vi "read_weather_station.vi"() -> ()   [LabVIEW 2011]
panel:
  out "Deque error":errorcluster
  out "DataSocket error":errorcluster
  out "# Sent Data":u64
  out "Solar position (elevation)":string
  out "Solar position (azimuth)":string
  out "Dew point temperature":string
  out "Absolute air humidity":string
  out "Relative air humidity":string
  out "Relative air pressure":string
  out "Absolute air pressure":string
  out "Wind direction":string
  out "Wind velocity":string
  out "Precipiation":string
  out "Outside temperature":string
  out "Global radiation":string
  out "Twilight":string
  out "Brigthness, western direction":string
  out "Brigthness, southern direction":string
  out "Brigthness, eastern direction":string
  out "Brigthness, northen direction":string
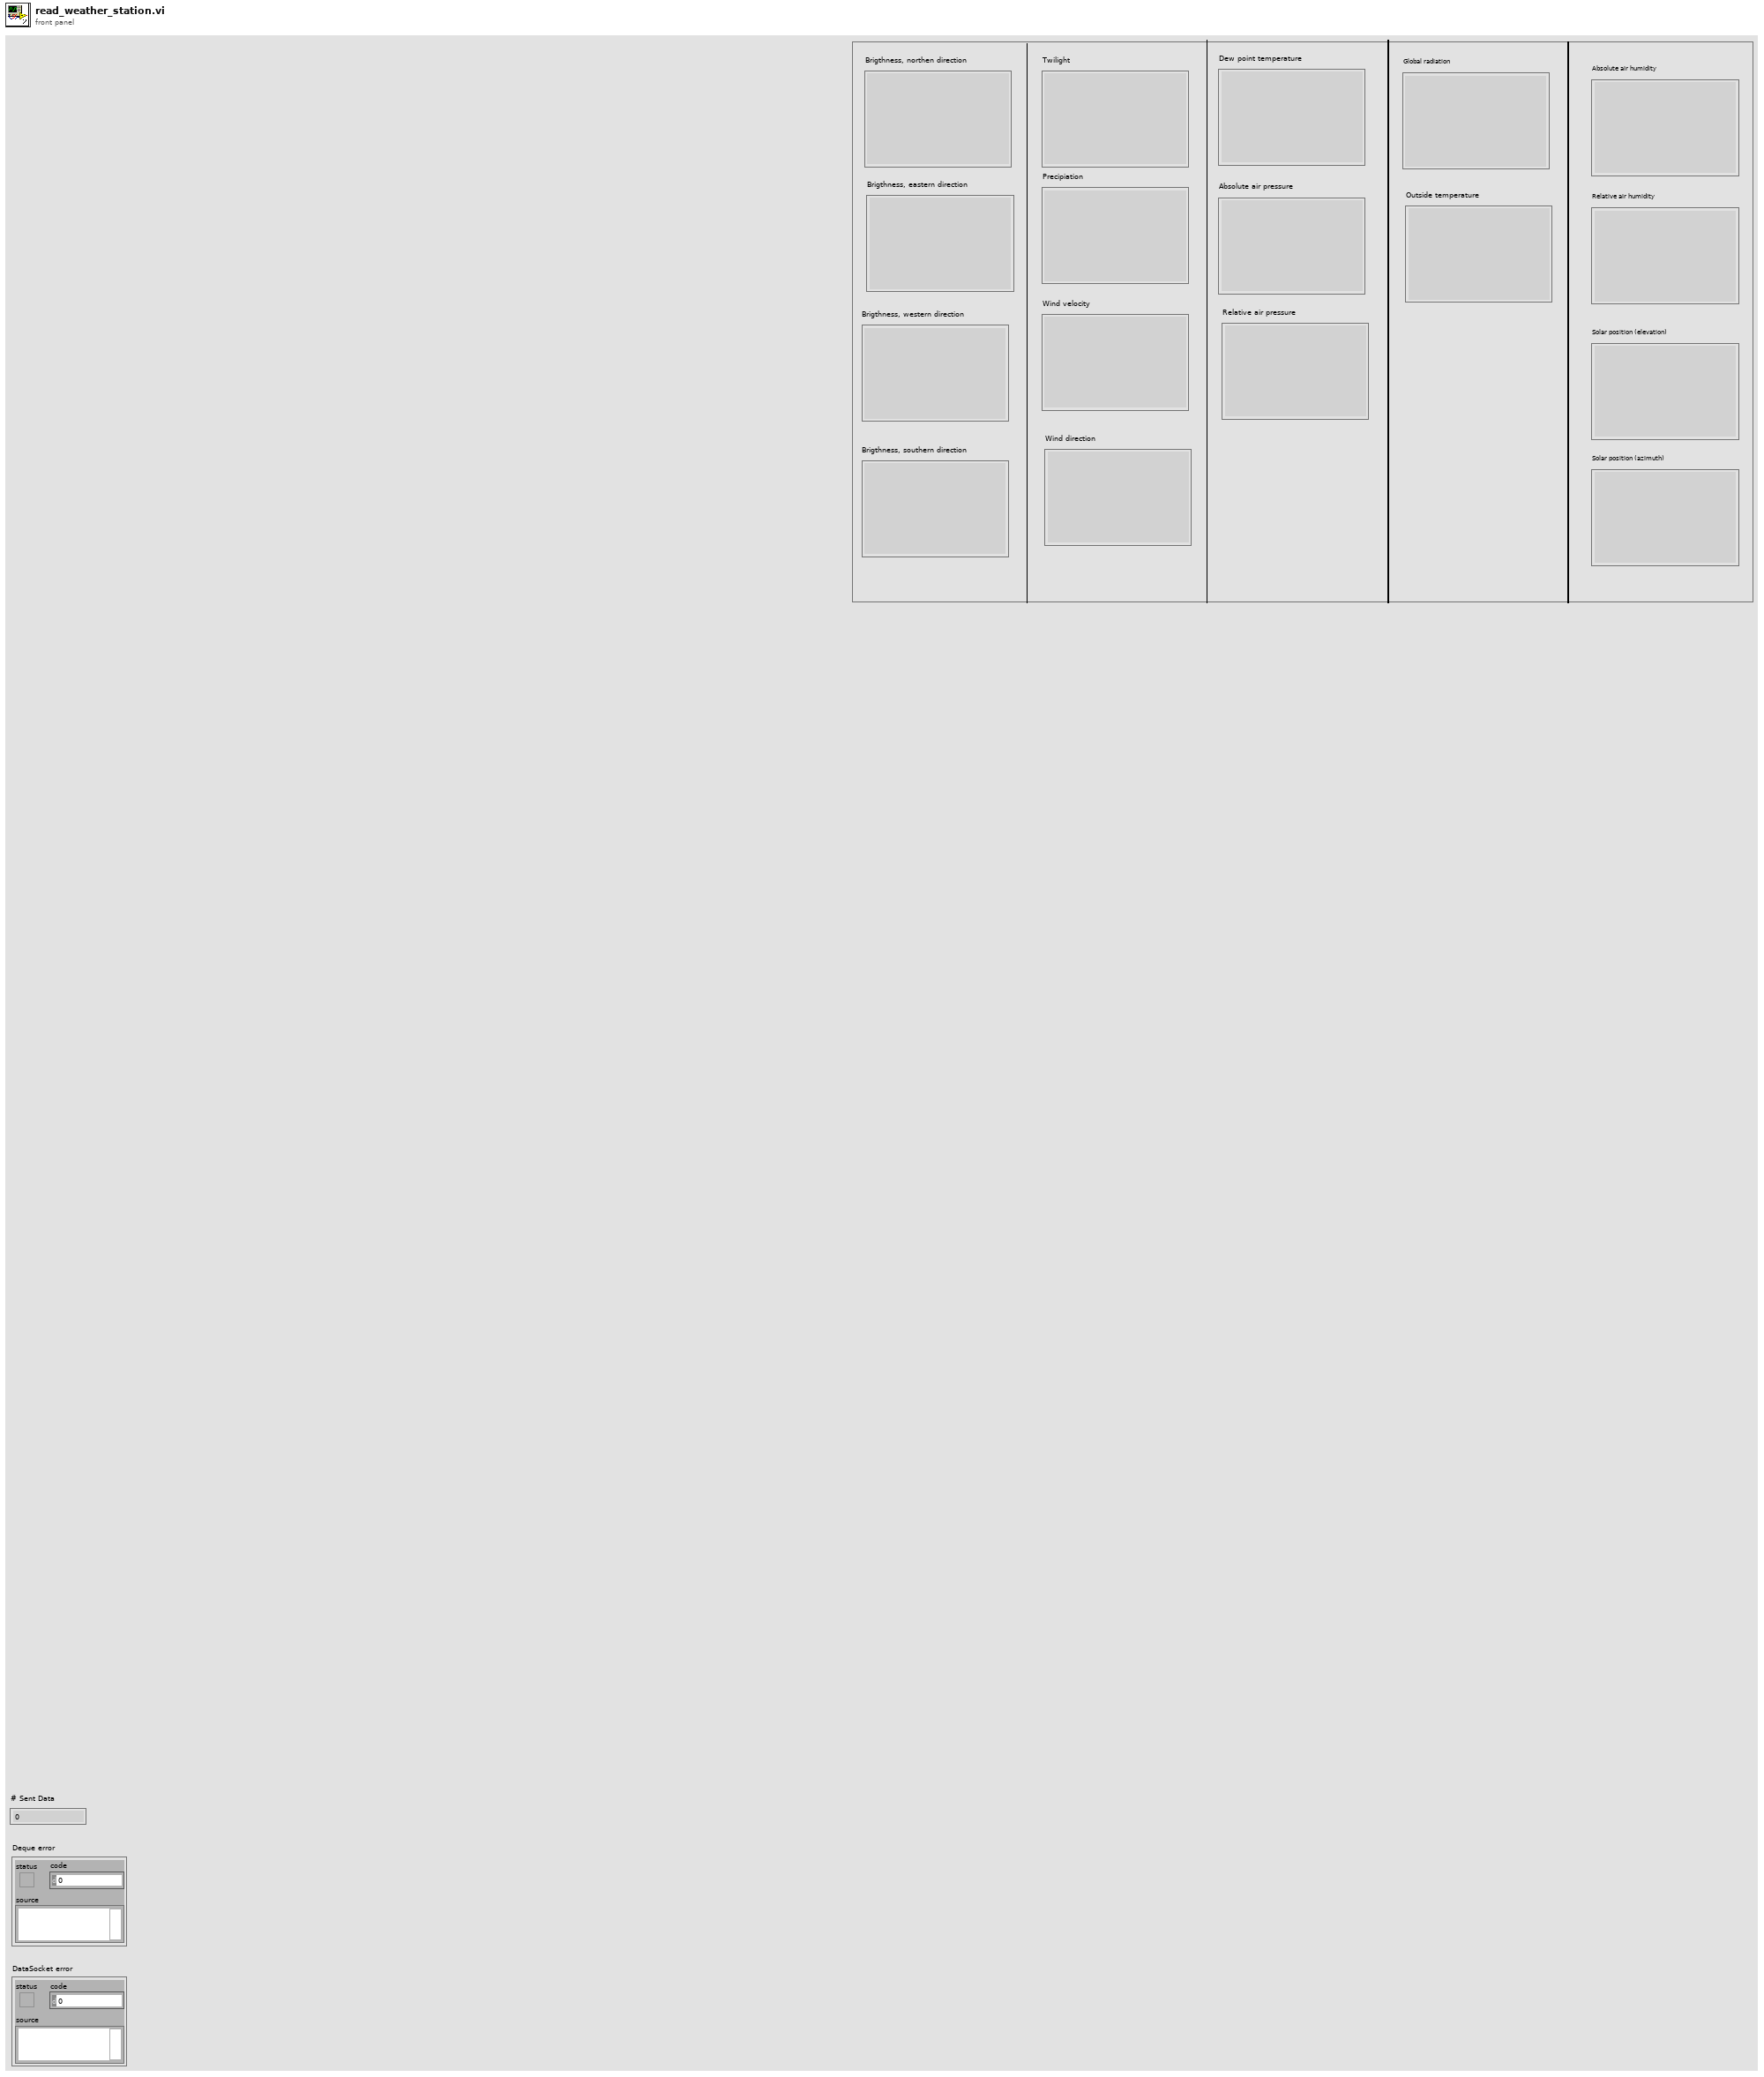
[diagram p1: front panel]
types:
  T1 = enum16{"Read", "Write", "ReadWrite", "BufferedRead", "BufferedReadWrite"}
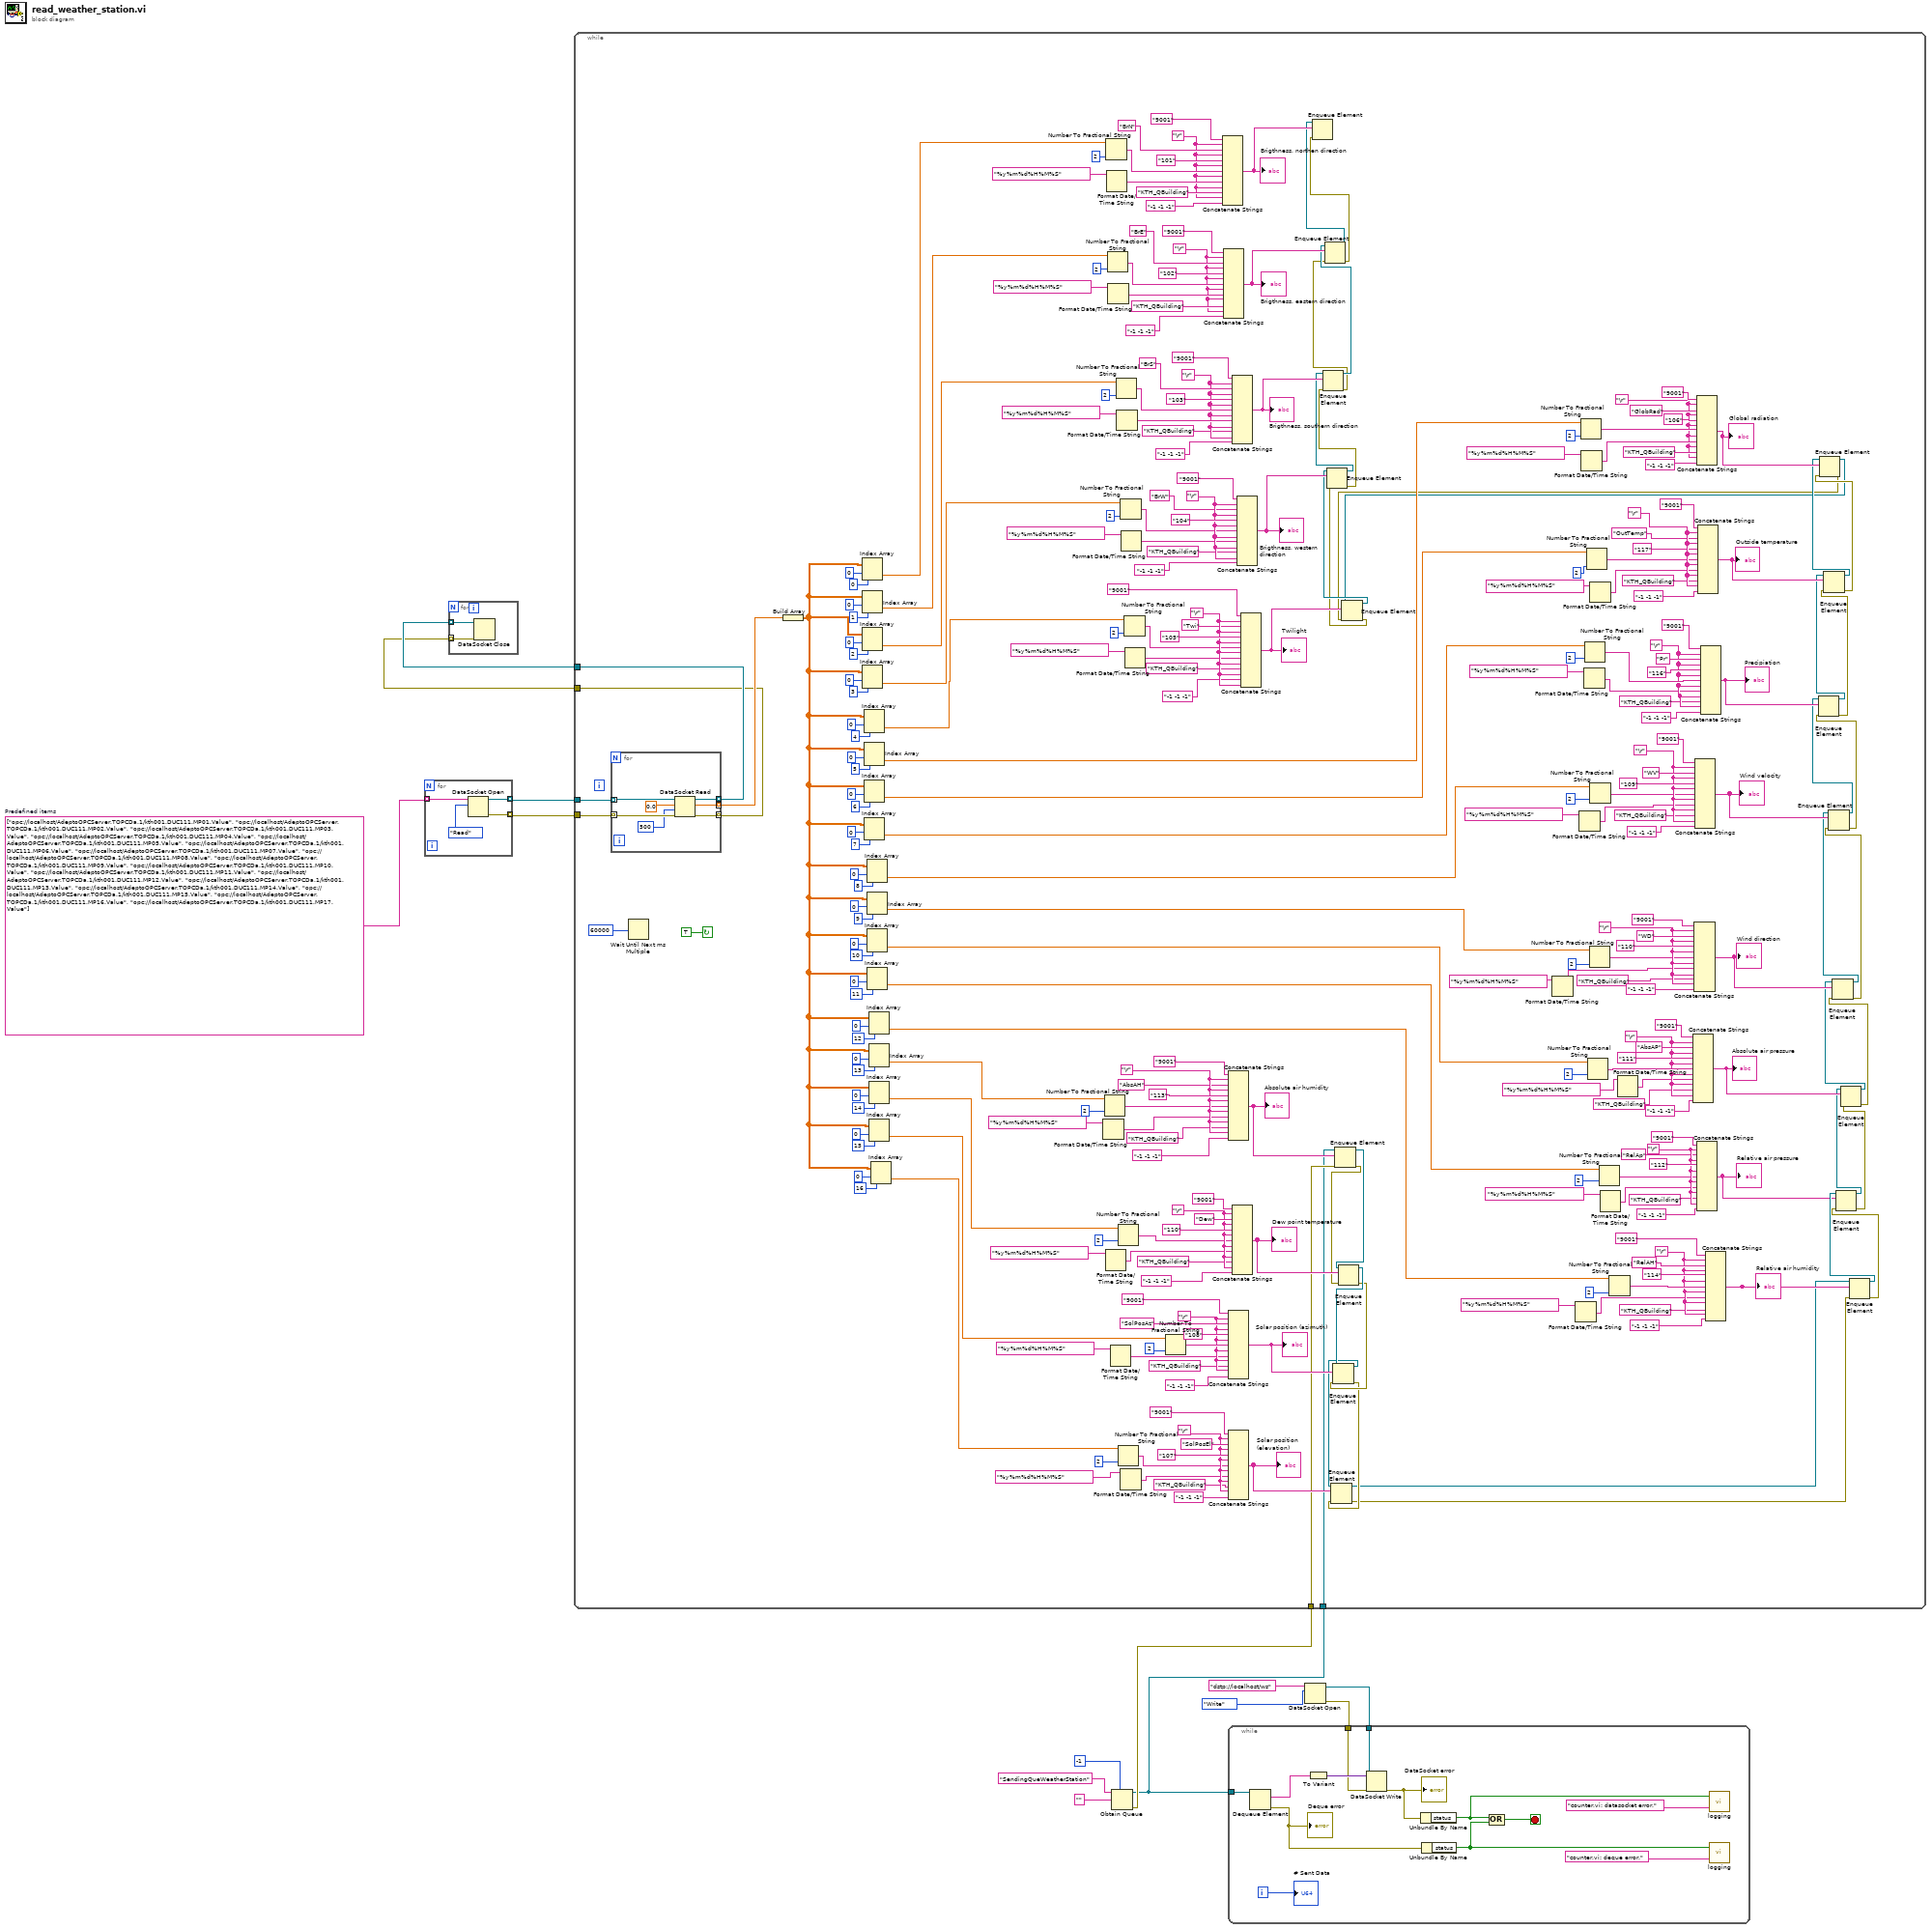
[diagram p0: block diagram]
diagram:
  w14 = string[] ["opc://localhost/AdeptoOPCServer.TOPCDa.1/kth001.DUC111.MP01.Value", "opc://localhost/AdeptoOPCServer.TOPCDa.1/kth001.DUC111.MP02.Value", "opc://localhost/AdeptoOPCServer.TOPCDa.1/kth001.DUC111.MP03.Value", "opc://localhost/AdeptoOPCServer.TOPCDa.1/kth001.DUC111.MP04.Value", "opc://localhost/AdeptoOPCServer.TOPCDa.1/kth001.DUC111.MP05.Value", "opc://localhost/AdeptoOPCServer.TOPCDa.1/kth001.DUC111.MP06.Value", "opc://localhost/AdeptoOPCServer.TOPCDa.1/kth001.DUC111.MP07.Value", "opc://localhost/AdeptoOPCServer.TOPCDa.1/kth001.DUC111.MP08.Value", "opc://localhost/AdeptoOPCServer.TOPCDa.1/kth001.DUC111.MP09.Value", "opc://localhost/AdeptoOPCServer.TOPCDa.1/kth001.DUC111.MP10.Value", "opc://localhost/AdeptoOPCServer.TOPCDa.1/kth001.DUC111.MP11.Value", "opc://localhost/AdeptoOPCServer.TOPCDa.1/kth001.DUC111.MP12.Value", "opc://localhost/AdeptoOPCServer.TOPCDa.1/kth001.DUC111.MP13.Value", "opc://localhost/AdeptoOPCServer.TOPCDa.1/kth001.DUC111.MP14.Value", "opc://localhost/AdeptoOPCServer.TOPCDa.1/kth001.DUC111.MP15.Value", "opc://localhost/AdeptoOPCServer.TOPCDa.1/kth001.DUC111.MP16.Value", "opc://localhost/AdeptoOPCServer.TOPCDa.1/kth001.DUC111.MP17.Value"]  # Predefined items
  n1 = for {
    tunnel: w14 -> [w18] mode=indexing
    tunnel: [w17] -> w13 mode=indexing
    tunnel: [w16] -> w12 mode=indexing
    n2 = DataSocket Open(10:T1."Read" ("mode"), 11:w18) -> (0:w16:errorcluster, 3:w17:refnum<k13>)  [unwired: 1 in, 1 out]
  }
  n3 = Obtain Queue(max queue size (-1, unlimited)=-1, name (unnamed)="SendingQueWeatherStation", element data type="") -> (queue out=w1:refnum<queue>, error out=w2:errorcluster)  [unwired: 2 in, 1 out]
  n4 = while {
    tunnel: w13 -> [w295]
    tunnel: w12 -> [w294]
    tunnel: [w292] -> w11
    tunnel: [w291] -> w10
    tunnel: w2 -> [w20]
    tunnel: w1 -> [w19]
    stop <- TRUE continue-if-true
    w74 = "\r"
    w79 = "\r"
    w86 = "\r"
    w93 = "\r"
    w97 = "\r"
    w105 = "\r"
    w109 = "\r"
    w116 = "\r"
    w123 = "\r"
    w128 = "\r"
    w137 = "\r"
    w138 = "\r"
    w150 = "\r"
    w156 = "\r"
    w159 = "\r"
    w164 = "\r"
    w170 = "\r"
    n5 = for {
      tunnel: w295 -> [w303] mode=indexing
      tunnel: [w305] -> w292 mode=indexing
      tunnel: w294 -> [w302] mode=indexing
      tunnel: [w300] -> w293 mode=indexing
      tunnel: [w304] -> w291 mode=indexing
      n6 = DataSocket Read(8:w302, 9:500 ("ms timeout (10000)"), 10:0.0, 11:w303) -> (0:w304:errorcluster, 2:w300:dbl, 3:w305:refnum<k13>)  [unwired: 5 out]
    }
    n7 = Wait Until Next ms Multiple(millisecond multiple=u32 60000) -> ()  [unwired: 1 out]
    n8 = Build Array(w293) -> (w238:dbl[][])
    n9 = Index Array(array=w238, index (row)=0, index (col)=0 ("disabled index (col)")) -> (element=w282:dbl)
    n10 = Index Array(array=w238, index (row)=0, index (col)=1 ("disabled index (col)")) -> (element=w274:dbl)
    n11 = Index Array(array=w238, index (row)=0, index (col)=2 ("disabled index (col)")) -> (element=w224:dbl)
    n12 = Index Array(array=w238, index (row)=0, index (col)=3 ("disabled index (col)")) -> (element=w265:dbl)
    n13 = Index Array(array=w238, index (row)=0, index (col)=4 ("disabled index (col)")) -> (element=w233:dbl)
    n14 = Index Array(array=w238, index (row)=0, index (col)=5 ("disabled index (col)")) -> (element=w226:dbl)
    n15 = Index Array(array=w238, index (row)=0, index (col)=6 ("disabled index (col)")) -> (element=w225:dbl)
    n16 = Index Array(array=w238, index (row)=0, index (col)=7 ("disabled index (col)")) -> (element=w219:dbl)
    n17 = Index Array(array=w238, index (row)=0, index (col)=8 ("disabled index (col)")) -> (element=w214:dbl)
    n18 = Index Array(array=w238, index (row)=0, index (col)=9 ("disabled index (col)")) -> (element=w210:dbl)
    n19 = Index Array(array=w238, index (row)=0, index (col)=10 ("disabled index (col)")) -> (element=w205:dbl)
    n20 = Index Array(array=w238, index (row)=0, index (col)=11 ("disabled index (col)")) -> (element=w200:dbl)
    n21 = Index Array(array=w238, index (row)=0, index (col)=12 ("disabled index (col)")) -> (element=w195:dbl)
    n22 = Index Array(array=w238, index (row)=0, index (col)=13 ("disabled index (col)")) -> (element=w190:dbl)
    n23 = Index Array(array=w238, index (row)=0, index (col)=14 ("disabled index (col)")) -> (element=w186:dbl)
    n24 = Index Array(array=w238, index (row)=0, index (col)=15 ("disabled index (col)")) -> (element=w175:dbl)
    n25 = Index Array(array=w238, index (row)=0, index (col)=16 ("disabled index (col)")) -> (element=w176:dbl)
    n26 = Format Date/Time String(time format string (%c)="%y%m%d%H%M%S") -> (date/time string=w90:string)  [unwired: 2 in]
    n27 = Number To Fractional String(number=w190, precision (6)=i16 2) -> (F-format string=w91:string)  [unwired: 2 in]
    n28 = Format Date/Time String(time format string (%c)="%y%m%d%H%M%S") -> (date/time string=w84:string)  [unwired: 2 in]
    n29 = Number To Fractional String(number=w282, precision (6)=i16 2) -> (F-format string=w173:string)  [unwired: 2 in]
    n30 = Format Date/Time String(time format string (%c)="%y%m%d%H%M%S") -> (date/time string=w172:string)  [unwired: 2 in]
    n31 = Number To Fractional String(number=w274, precision (6)=i16 2) -> (F-format string=w167:string)  [unwired: 2 in]
    n32 = Format Date/Time String(time format string (%c)="%y%m%d%H%M%S") -> (date/time string=w166:string)  [unwired: 2 in]
    n33 = Format Date/Time String(time format string (%c)="%y%m%d%H%M%S") -> (date/time string=w78:string)  [unwired: 2 in]
    n34 = Number To Fractional String(number=w224, precision (6)=i16 2) -> (F-format string=w161:string)  [unwired: 2 in]
    n35 = Format Date/Time String(time format string (%c)="%y%m%d%H%M%S") -> (date/time string=w160:string)  [unwired: 2 in]
    n36 = Number To Fractional String(number=w186, precision (6)=i16 2) -> (F-format string=w85:string)  [unwired: 2 in]
    n37 = Number To Fractional String(number=w176, precision (6)=i16 2) -> (F-format string=w73:string)  [unwired: 2 in]
    n38 = Number To Fractional String(number=w265, precision (6)=i16 2) -> (F-format string=w154:string)  [unwired: 2 in]
    n39 = Format Date/Time String(time format string (%c)="%y%m%d%H%M%S") -> (date/time string=w72:string)  [unwired: 2 in]
    n40 = Format Date/Time String(time format string (%c)="%y%m%d%H%M%S") -> (date/time string=w153:string)  [unwired: 2 in]
    n41 = Number To Fractional String(number=w233, precision (6)=i16 2) -> (F-format string=w148:string)  [unwired: 2 in]
    n42 = Format Date/Time String(time format string (%c)="%y%m%d%H%M%S") -> (date/time string=w147:string)  [unwired: 2 in]
    n43 = Number To Fractional String(number=w175, precision (6)=i16 2) -> (F-format string=w80:string)  [unwired: 2 in]
    n44 = Concatenate Strings("9001" ("string"), w170, "BrN" ("string"), w170, "101" ("string"), w170, w173, w170, w172, w170, "KTH_QBuilding" ("string"), w170, "-1 -1 -1" ("string")) -> (w46:string)
    "Brigthness, northen direction" <- w46
    n45 = Concatenate Strings("9001" ("string"), w164, "BrE" ("string"), w164, "102" ("string"), w164, w167, w164, w166, w164, "KTH_QBuilding" ("string"), w164, "-1 -1 -1" ("string")) -> (w47:string)
    "Brigthness, eastern direction" <- w47
    n46 = Concatenate Strings("9001" ("string"), w93, "AbsAH" ("string"), w93, "113" ("string"), w93, w91, w93, w90, w93, "KTH_QBuilding" ("string"), w93, "-1 -1 -1" ("string")) -> (w68:string)
    "Absolute air humidity" <- w68
    n47 = Concatenate Strings("9001" ("string"), w79, "SolPosAz" ("string"), w79, "108" ("string"), w79, w80, w79, w78, w79, "KTH_QBuilding" ("string"), w79, "-1 -1 -1" ("string")) -> (w66:string)
    "Solar position (azimuth)" <- w66
    n48 = Concatenate Strings("9001" ("string"), w74, "SolPosEl" ("string"), w74, "107" ("string"), w74, w73, w74, w72, w74, "KTH_QBuilding" ("string"), w74, "-1 -1 -1" ("string")) -> (w69:string)
    "Solar position (elevation)" <- w69
    n49 = Concatenate Strings("9001" ("string"), w159, "BrS" ("string"), w159, "103" ("string"), w159, w161, w159, w160, w159, "KTH_QBuilding" ("string"), w159, "-1 -1 -1" ("string")) -> (w48:string)
    "Brigthness, southern direction" <- w48
    n50 = Concatenate Strings("9001" ("string"), w86, "Dew" ("string"), w86, "110" ("string"), w86, w85, w86, w84, w86, "KTH_QBuilding" ("string"), w86, "-1 -1 -1" ("string")) -> (w67:string)
    "Dew point temperature" <- w67
    n51 = Concatenate Strings("9001" ("string"), w156, "BrW" ("string"), w156, "104" ("string"), w156, w154, w156, w153, w156, "KTH_QBuilding" ("string"), w156, "-1 -1 -1" ("string")) -> (w49:string)
    "Brigthness, western direction" <- w49
    n52 = Concatenate Strings("9001" ("string"), w150, "Twi" ("string"), w150, "105" ("string"), w150, w148, w150, w147, w150, "KTH_QBuilding" ("string"), w150, "-1 -1 -1" ("string"), w150) -> (w50:string)
    "Twilight" <- w50
    n53 = Enqueue Element(queue=w19, element=w68, error in (no error)=w20) -> (queue out=w28:refnum<queue>, error out=w27:errorcluster)  [unwired: 1 in, 1 out]
    n54 = Enqueue Element(queue=w28, element=w67, error in (no error)=w27) -> (queue out=w26:refnum<queue>, error out=w25:errorcluster)  [unwired: 1 in, 1 out]
    n55 = Enqueue Element(queue=w26, element=w66, error in (no error)=w25) -> (queue out=w24:refnum<queue>, error out=w23:errorcluster)  [unwired: 1 in, 1 out]
    n56 = Enqueue Element(queue=w24, element=w69, error in (no error)=w23) -> (queue out=w21:refnum<queue>, error out=w22:errorcluster)  [unwired: 1 in, 1 out]
    n57 = Format Date/Time String(time format string (%c)="%y%m%d%H%M%S") -> (date/time string=w114:string)  [unwired: 2 in]
    n58 = Format Date/Time String(time format string (%c)="%y%m%d%H%M%S") -> (date/time string=w96:string)  [unwired: 2 in]
    n59 = Format Date/Time String(time format string (%c)="%y%m%d%H%M%S") -> (date/time string=w121:string)  [unwired: 2 in]
    n60 = Number To Fractional String(number=w226, precision (6)=i16 2) -> (F-format string=w142:string)  [unwired: 2 in]
    n61 = Format Date/Time String(time format string (%c)="%y%m%d%H%M%S") -> (date/time string=w141:string)  [unwired: 2 in]
    n62 = Format Date/Time String(time format string (%c)="%y%m%d%H%M%S") -> (date/time string=w127:string)  [unwired: 2 in]
    n63 = Number To Fractional String(number=w219, precision (6)=i16 2) -> (F-format string=w129:string)  [unwired: 2 in]
    n64 = Number To Fractional String(number=w225, precision (6)=i16 2) -> (F-format string=w134:string)  [unwired: 2 in]
    n65 = Number To Fractional String(number=w205, precision (6)=i16 2) -> (F-format string=w110:string)  [unwired: 2 in]
    n66 = Number To Fractional String(number=w210, precision (6)=i16 2) -> (F-format string=w115:string)  [unwired: 2 in]
    n67 = Format Date/Time String(time format string (%c)="%y%m%d%H%M%S") -> (date/time string=w133:string)  [unwired: 2 in]
    n68 = Number To Fractional String(number=w214, precision (6)=i16 2) -> (F-format string=w122:string)  [unwired: 2 in]
    n69 = Number To Fractional String(number=w200, precision (6)=i16 2) -> (F-format string=w103:string)  [unwired: 2 in]
    n70 = Format Date/Time String(time format string (%c)="%y%m%d%H%M%S") -> (date/time string=w102:string)  [unwired: 2 in]
    n71 = Number To Fractional String(number=w195, precision (6)=i16 2) -> (F-format string=w98:string)  [unwired: 2 in]
    n72 = Format Date/Time String(time format string (%c)="%y%m%d%H%M%S") -> (date/time string=w108:string)  [unwired: 2 in]
    n73 = Concatenate Strings("9001" ("string"), w109, "AbsAP" ("string"), w109, "111" ("string"), w109, w110, w109, w108, w109, "KTH_QBuilding" ("string"), w109, "-1 -1 -1" ("string")) -> (w62:string)
    "Absolute air pressure" <- w62
    n74 = Concatenate Strings("9001" ("string"), w116, "WD" ("string"), w116, "110" ("string"), w116, w115, w116, w114, w116, "KTH_QBuilding" ("string"), w116, "-1 -1 -1" ("string")) -> (w61:string)
    "Wind direction" <- w61
    n75 = Concatenate Strings("9001" ("string"), w123, "WV" ("string"), w123, "109" ("string"), w123, w122, w123, w121, w123, "KTH_QBuilding" ("string"), w123, "-1 -1 -1" ("string")) -> (w60:string)
    "Wind velocity" <- w60
    n76 = Concatenate Strings("9001" ("string"), w138, "GlobRad" ("string"), w138, "106" ("string"), w138, w142, w138, w141, w138, "KTH_QBuilding" ("string"), w138, "-1 -1 -1" ("string")) -> (w57:string)
    "Global radiation" <- w57
    n77 = Concatenate Strings("9001" ("string"), w105, "RelAp" ("string"), w105, "112" ("string"), w105, w103, w105, w102, w105, "KTH_QBuilding" ("string"), w105, "-1 -1 -1" ("string")) -> (w63:string)
    "Relative air pressure" <- w63
    n78 = Concatenate Strings("9001" ("string"), w137, "OutTemp" ("string"), w137, "117" ("string"), w137, w134, w137, w133, w137, "KTH_QBuilding" ("string"), w137, "-1 -1 -1" ("string")) -> (w58:string)
    "Outside temperature" <- w58
    n79 = Concatenate Strings("9001" ("string"), w128, "Pr" ("string"), w128, "116" ("string"), w128, w129, w128, w127, w128, "KTH_QBuilding" ("string"), w128, "-1 -1 -1" ("string")) -> (w59:string)
    "Precipiation" <- w59
    n80 = Concatenate Strings("9001" ("string"), w97, "RelAH" ("string"), w97, "114" ("string"), w97, w98, w97, w96, w97, "KTH_QBuilding" ("string"), w97, "-1 -1 -1" ("string")) -> (w64:string)
    "Relative air humidity" <- w64
    n81 = Enqueue Element(queue=w21, element=w64, error in (no error)=w22) -> (queue out=w65:refnum<queue>, error out=w41:errorcluster)  [unwired: 1 in, 1 out]
    n82 = Enqueue Element(queue=w65, element=w63, error in (no error)=w41) -> (queue out=w56:refnum<queue>, error out=w40:errorcluster)  [unwired: 1 in, 1 out]
    n83 = Enqueue Element(queue=w56, element=w62, error in (no error)=w40) -> (queue out=w55:refnum<queue>, error out=w39:errorcluster)  [unwired: 1 in, 1 out]
    n84 = Enqueue Element(queue=w55, element=w61, error in (no error)=w39) -> (queue out=w54:refnum<queue>, error out=w38:errorcluster)  [unwired: 1 in, 1 out]
    n85 = Enqueue Element(queue=w54, element=w60, error in (no error)=w38) -> (queue out=w53:refnum<queue>, error out=w37:errorcluster)  [unwired: 1 in, 1 out]
    n86 = Enqueue Element(queue=w53, element=w59, error in (no error)=w37) -> (queue out=w52:refnum<queue>, error out=w36:errorcluster)  [unwired: 1 in, 1 out]
    n87 = Enqueue Element(queue=w52, element=w58, error in (no error)=w36) -> (queue out=w51:refnum<queue>, error out=w35:errorcluster)  [unwired: 1 in, 1 out]
    n88 = Enqueue Element(queue=w51, element=w57, error in (no error)=w35) -> (queue out=w34:refnum<queue>, error out=w33:errorcluster)  [unwired: 1 in, 1 out]
    n89 = Enqueue Element(queue=w34, element=w50, error in (no error)=w33) -> (queue out=w45:refnum<queue>, error out=w32:errorcluster)  [unwired: 1 in, 1 out]
    n90 = Enqueue Element(queue=w45, element=w49, error in (no error)=w32) -> (queue out=w44:refnum<queue>, error out=w31:errorcluster)  [unwired: 1 in, 1 out]
    n91 = Enqueue Element(queue=w44, element=w48, error in (no error)=w31) -> (queue out=w43:refnum<queue>, error out=w30:errorcluster)  [unwired: 1 in, 1 out]
    n92 = Enqueue Element(queue=w43, element=w47, error in (no error)=w30) -> (queue out=w42:refnum<queue>, error out=w29:errorcluster)  [unwired: 1 in, 1 out]
    n93 = Enqueue Element(queue=w42, element=w46, error in (no error)=w29) -> ()  [unwired: 1 in, 3 out]
  }
  n94 = for {
    tunnel: w11 -> [w307] mode=indexing
    tunnel: w10 -> [w306] mode=indexing
    n95 = DataSocket Close(8:w306, 11:w307) -> ()  [unwired: 3 out]
  }
  n96 = DataSocket Open(10:T1."Write" ("mode"), 11:"dstp://localhost/ws" ("URL 3")) -> (0:w4:errorcluster, 3:w5:refnum<k13>)  [unwired: 2 in]
  n97 = while {
    tunnel: w1 -> [w320]
    tunnel: w5 -> [w319]
    tunnel: w4 -> [w314]
    i -> [w312]
    stop <- w313 stop-if-true
    n98 = Dequeue Element(queue=w320) -> (element=w317:string, error out=w316:errorcluster)  [unwired: 2 in, 2 out]
    "Deque error" <- w316
    n99 = To Variant(anything=w317) -> (Variant=w318:variant)
    n100 = DataSocket Write(8:w314, 10:w318, 11:w319) -> (0:w315:errorcluster)  [unwired: 3 out]
    "DataSocket error" <- w315
    n101 = Unbundle By Name(w315) -> ("status"=w309:bool)
    n102 = Unbundle By Name(w316) -> ("status"=w308:bool)
    n103 = Compound Arithmetic op=OR(w309, w308) -> (w313:bool)
    n104 = call "logging.vi"("data"="counter.vi: datasocket error.", "Boolean"=w309) -> ()  [unwired: 1 in]
    n105 = call "logging.vi"("data"="counter.vi: deque error.", "Boolean"=w308) -> ()  [unwired: 1 in]
    "# Sent Data" <- w312
  }
